vi "MT_GET_100.vi"(8 "Use checksum":bool, 11 "read buffer":string) -> (0 "MT check sum":u8, 1 "sample counter":i16, 2 "MT_DATA":sgl[](array[numeric])=[0.0, 0.0, -9.81, 0.0, 0.0, 0.0, 0.2, 0.0, 0.9], 4 "MT_BITS":u8[](array[numeric]))   [LabVIEW 2014]
uses:
  <vilib>/imath/engines/lvmath2/RunTimeEngine/BuiltInFunctions/length/NIMS_length(GV).vi
  <instcachedir>/0/NIMS_length(GV)_08A3D13377FD4E4B96F5795FBF3698FA.lvgen/NIMS_length(GV)_08A3D13377FD4E4B96F5795FBF3698FA_003.vi
  <vilib>/imath/engines/lvmath2/RunTimeEngine/RangeToken/NIMS_Range_R2 - Integer.vi
  <instcachedir>/0/NIMS_Range_R2 - Integer_2D1304BAF97744E0A293025746CBADFC.lvgen/NIMS_Range_R2 - Integer_2D1304BAF97744E0A293025746CBADFC_000.vi
  <vilib>/imath/engines/lvmath2/RunTimeEngine/CommandStatement/MC_CommandStatement_break.vi
  <vilib>/imath/engines/lvmath2/RunTimeEngine/IndexRead/NIMS V(S).vi
  <instcachedir>/0/NIMS V(S)_0488751826AF41519A22953C041130DC.lvgen/NIMS V(S)_0488751826AF41519A22953C041130DC_003.vi
  <vilib>/imathl/engines/lvmath/Functions/Error Handling/Create Error.vi
  <vilib>/imath/engines/lvmath2/RunTimeEngine/BuiltInFunctions/mod/NIMS_mod_no_size_check.vi
  <instcachedir>/0/NIMS_mod_no_size_check_5393E3382FD241D281EEB71DA286C65B.lvgen/NIMS_mod_no_size_check_5393E3382FD241D281EEB71DA286C65B_008.vi
  <vilib>/imath/engines/lvmath2/RunTimeEngine/BuiltInFunctions/uint8/NIMS_uint8(int).vi
  <instcachedir>/0/NIMS_uint8(int)_9D6EF81F86254677BB00410F9E5C6A1D.lvgen/NIMS_uint8(int)_9D6EF81F86254677BB00410F9E5C6A1D_000.vi
  <vilib>/imath/engines/lvmath2/RunTimeEngine/NodeEndStatement/NIMS_NodeEndStatement_Output.vi
  <instcachedir>/0/NIMS_NodeEndStatement_Output_53EC0D466D134D7ABD903AC30B43404B.lvgen/NIMS_NodeEndStatement_Output_53EC0D466D134D7ABD903AC30B43404B_013.vi
  <instcachedir>/0/NIMS_NodeEndStatement_Output_53EC0D466D134D7ABD903AC30B43404B.lvgen/NIMS_NodeEndStatement_Output_53EC0D466D134D7ABD903AC30B43404B_012.vi
  <vilib>/imath/engines/lvmath2/RunTimeEngine/ErrorHandling/NIMS_Finalize Error.vi
panel:
  out "New checksum":u8
  out "New checksum OK?":bool
  out "size(s)":i32
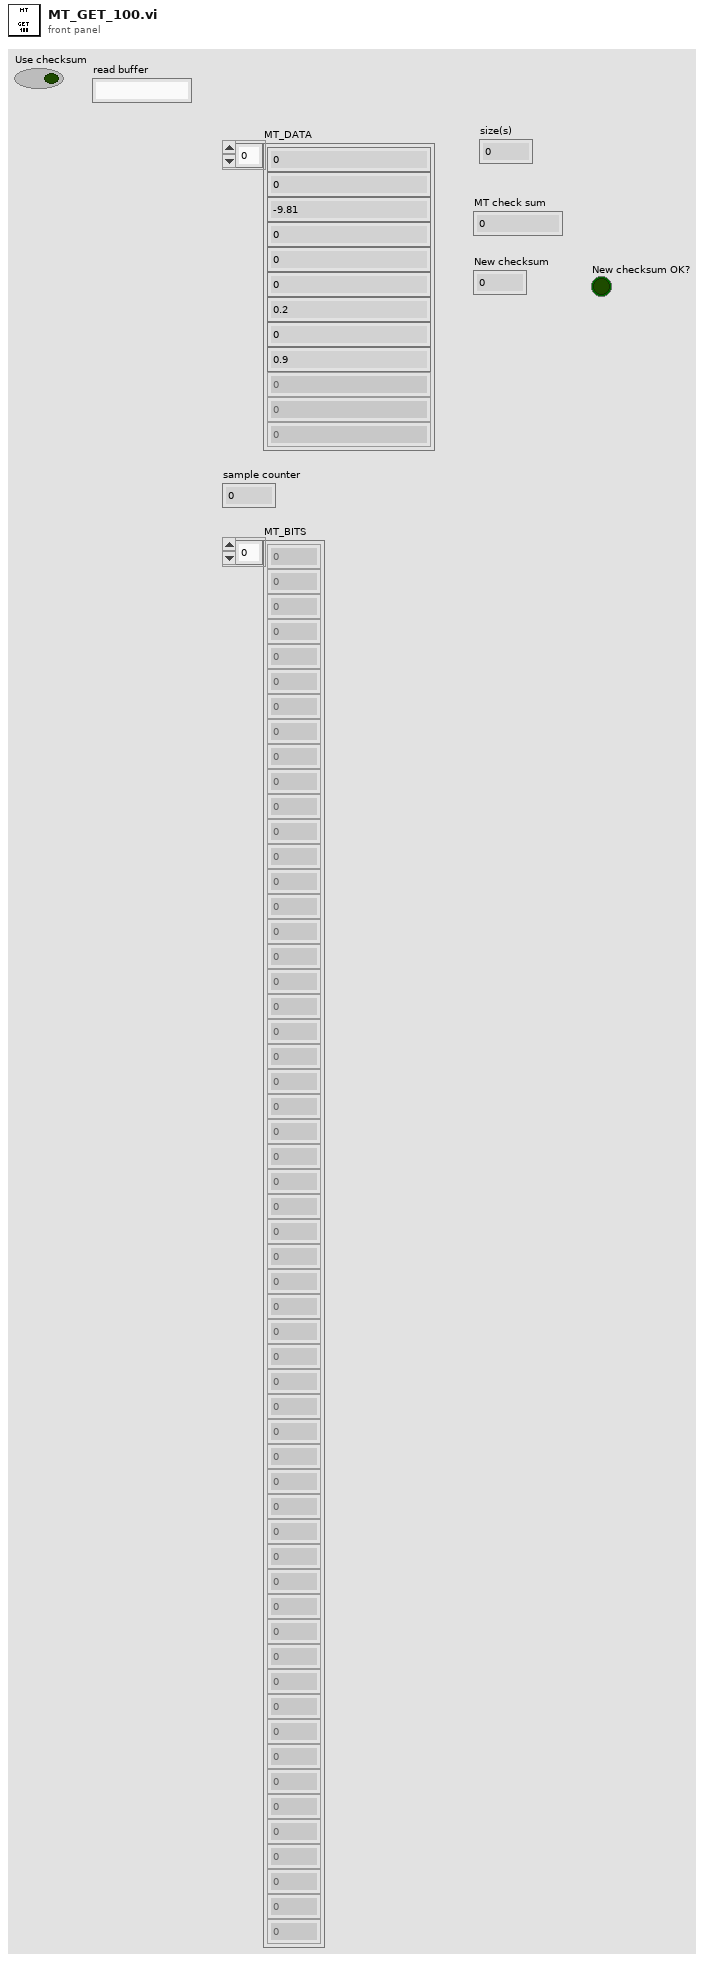
[diagram p1: front panel]
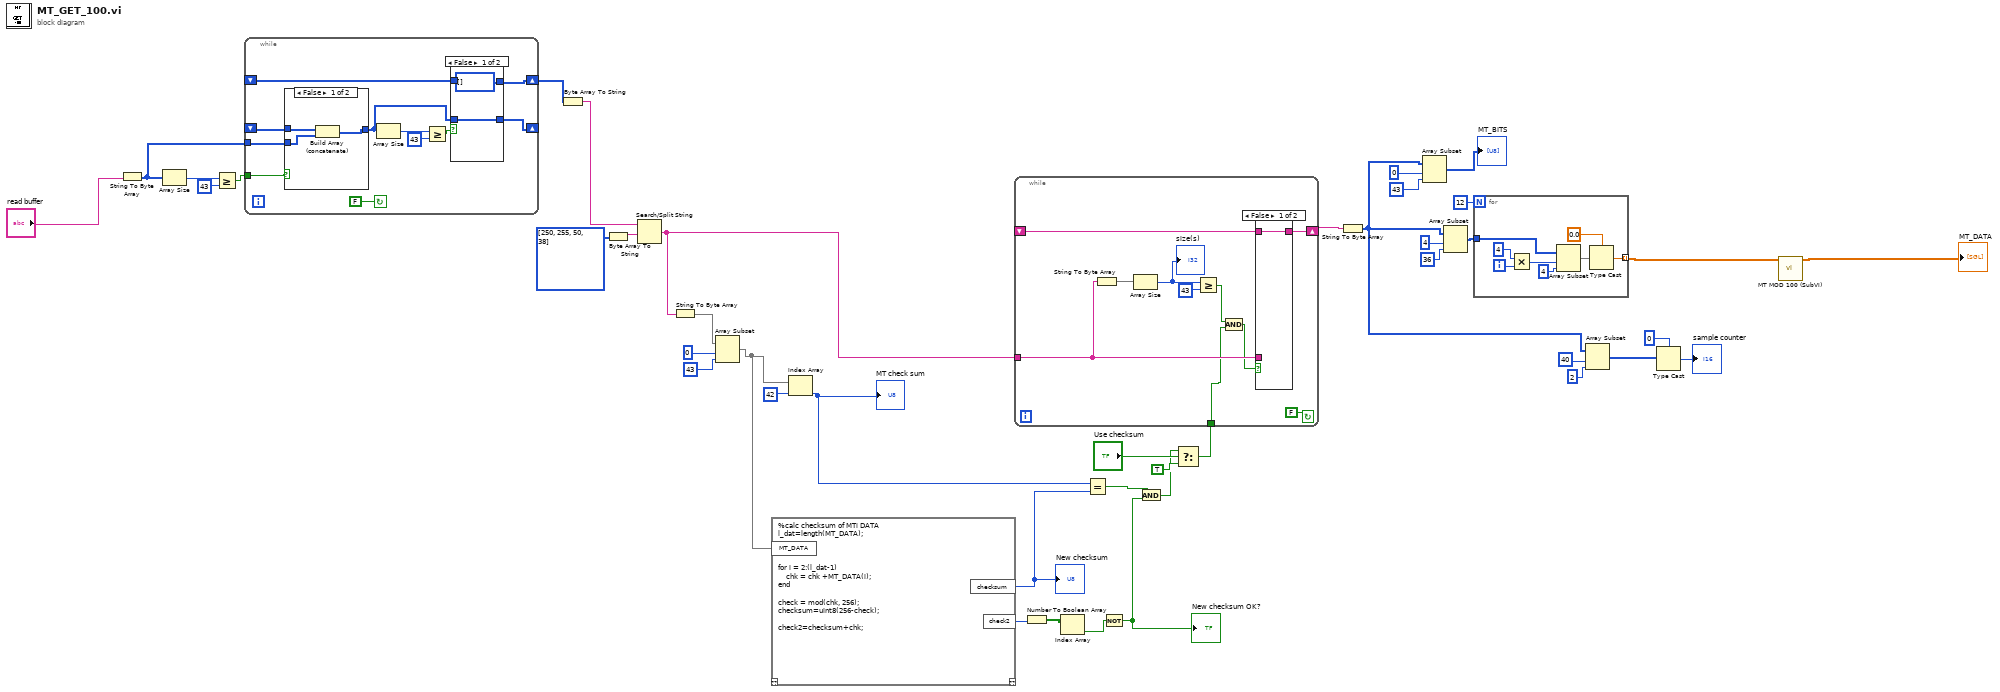
[diagram p0: block diagram]
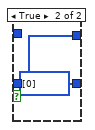
[diagram p2: hidden frame]
diagram:
  n1 = String To Byte Array(string="read buffer") -> (unsigned byte array=w3:u8[])
  n2 = Array Size(array=w3) -> (size(s)=w7:i32)
  n3 = Greater Or Equal?(x=w7, y=43) -> (x >= y?=w4:bool)
  n4 = while {
    shift-right: [w43] -> _
    shift-left: _ -> [w50]
    tunnel: w4 -> [w52]
    tunnel: w3 -> [w51]
    shift-right: [w45] -> w2
    shift-left: _ -> [w44]
    stop <- FALSE continue-if-true
    n5 = case shown="False" w52 {
      tunnel: w51 -> [w58 w61]
      tunnel: [w60 w61] -> w46
      tunnel: w50 -> [w59 _]
      frame False {
        n6 = Build Array (concatenate)(w59, w58) -> (w60:u8[])
      }
      frame True {
      }
    }
    n7 = Array Size(array=w46) -> (size(s)=w49:i32)
    n8 = Greater Or Equal?(x=w49, y=43) -> (x >= y?=w47:bool)
    n9 = case shown="False" w47 {
      tunnel: w46 -> [w55 w57]
      tunnel: [u8[] [] ("unsigned byte array") w57] -> w45
      tunnel: w44 -> [_ _]
      tunnel: [w55 u8[] [0] ("unsigned byte array")] -> w43
      frame False {
      }
      frame True {
      }
    }
  }
  n10 = Byte Array To String(unsigned byte array=w2) -> (string=w1:string)
  n11 = Byte Array To String(unsigned byte array=u8[] [250, 255, 50, 38]) -> (string=w42:string)
  n12 = Search/Split String(string=w1, search string/char (-)=w42) -> (match + rest of string=w27:string)  [unwired: 1 in, 2 out]
  n13 = String To Byte Array(string=w27) -> (unsigned byte array=w26:u8[])
  n14 = Array Subset(array=w26, index=0, length=43) -> (w25:u8[])
  n15 = mathscript code="%calc checksum of MTi DATA\nl_dat=length(MT_DATA);\n\nchk = 0;\n\nfor i = 2:(l_dat-1)\n    chk = chk +MT_DATA(i);\nend\n\ncheck = mod(chk, 256);\nchecksum=uint8(256-check);\n\ncheck2=checksum+chk;"("MT_DATA"=w25) -> ("checksum"=w23:u8, "check2"=w22:i32)  [unwired: 1 in, 1 out]
  "New checksum" <- w23
  n16 = Index Array(array=w25, index=42) -> (element=w24:u8)
  "MT check sum" <- w24
  n17 = Number To Boolean Array(number=w22) -> (Boolean array=w21:bool[])
  n18 = Index Array(array=w21) -> (element=w20:bool)  [unwired: 1 in]
  n19 = Equal?(x=w24, y=w23) -> (x = y?=w19:bool)
  n20 = Not(x=w20) -> (.not. x?=w18:bool)
  "New checksum OK?" <- w18
  n21 = And(x=w19, y=w18) -> (x .and. y?=w15:bool)
  n22 = Select(t=w15, s="Use checksum", f=TRUE) -> (s? t:f=w14:bool)
  n23 = while {
    tunnel: w27 -> [w67]
    shift-right: [w66] -> w29
    shift-left: _ -> [w65]
    tunnel: w14 -> [w62]
    stop <- FALSE continue-if-true
    n24 = String To Byte Array(string=w67) -> (unsigned byte array=w70:u8[])
    n25 = Array Size(array=w70) -> (size(s)=w69:i32)
    "size(s)" <- w69
    n26 = Greater Or Equal?(x=w69, y=43) -> (x >= y?=w64:bool)
    n27 = And(x=w64, y=w62) -> (x .and. y?=w63:bool)
    n28 = case shown="False" w63 {
      tunnel: w67 -> [_ w73]
      tunnel: [w72 w73] -> w66
      tunnel: w65 -> [w72 _]
      frame False {
      }
      frame True {
      }
    }
  }
  n29 = String To Byte Array(string=w29) -> (unsigned byte array=w9:u8[])
  n30 = Array Subset(array=w9, index=0, length=43) -> (→"MT_BITS":u8[])
  n31 = Array Subset(array=w9, index=4, length=36) -> (w34:u8[])
  n32 = for {
    N: 12 -> [_]
    tunnel: w34 -> [w76]
    tunnel: [w74] -> w13 mode=indexing
    i -> [w79]
    n33 = Multiply(x=4 ("index"), y=w79) -> (x*y=w77:i32)
    n34 = Array Subset(array=w76, index=w77, length=4) -> (w75:u8[])
    n35 = Type Cast(type=sgl 0.0, x=w75) -> (*(type *) &x=w74:sgl)
  }
  n36 = Array Subset(array=w9, index=40, length=2) -> (w39:u8[])
  n37 = Type Cast(type=i16 0, x=w39) -> (*(type *) &x=→"sample counter":i16)
  n38 = call "MT MOD 100 (SubVI).vi"("MT_DATA"=w13) -> ("MT_mod"=→"MT_DATA":dbl[])  [unwired: 10 in]
